vi "Spawn.vi"(6 "Start Direction":T1=enum."E", 8 "error in (no error)":errorcluster, 10 "Directive":T2, 11 "Mother in":refnum<class "Formics.lvclass">) -> (0 "error out":errorcluster, 2 "Replicated Class":refnum<class "Formics.lvclass">, 3 "Mother out":refnum<class "Formics.lvclass">)   [LabVIEW 2015, in "Formics.lvclass"]
uses:
  Formics.lvclass
  Formic Types.ctl
  Type Defs/Direction Enum.ctl
  Current Directive.ctl
  Formics.lvclass/Formics.ctl
  Coward Options.ctl
  Type Defs/SB Type Defs.lvlib
panel:
  in  "Spawn Direction":T1=enum."E"
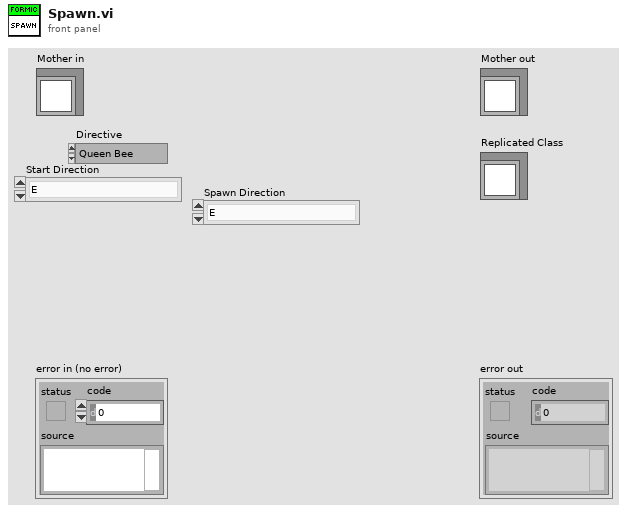
[diagram p1: front panel]
types:
  T1 = typedef "SB Type Defs.lvlib/Direction Enum.ctl" = enum16{"NW", "N", "NE", "E", "SE", "S", "SW", "W"}
  T2 = typedef "Formics.lvclass/Formic Types.ctl" = enum16{"Queen Bee", "Protector Bee", "Daughter Bee", "Worker Bee", "Coward"}
  T3 = typedef "Formics.lvclass/Current Directive.ctl" = enum16{"Queen", "Daughter", "Coward", "Migrate", "Line Up", "Protector", "Scout"}
  T4 = typedef "Formics.lvclass/Coward Options.ctl" = enum16{"Go", "Attack behind and continue", "Attack behind and recheck", "Move Back", "Check if still there"}
  T5 = typedef "Formics.lvclass/SquareStatus DVR.ctl" = refnum<data-value>
  T6 = typedef "Formics.lvclass/Kamikaze DVR.ctl" = refnum<data-value>
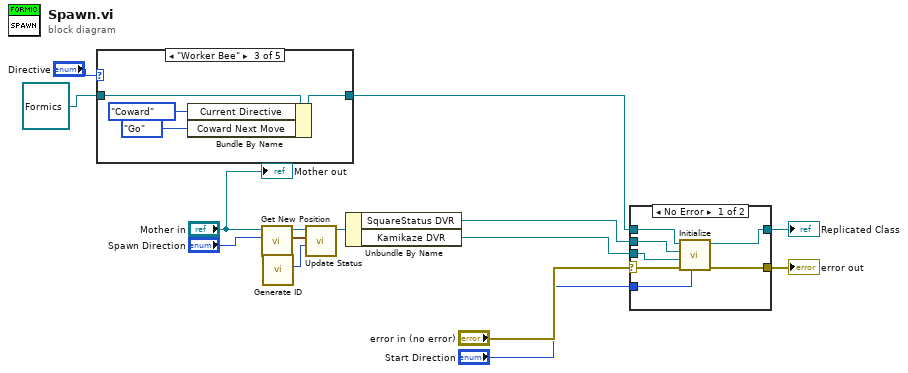
[diagram p0: block diagram]
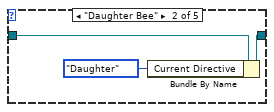
[diagram p3: hidden frame]
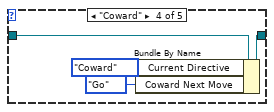
[diagram p4: hidden frame]
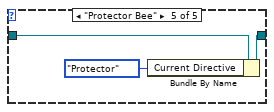
[diagram p5: hidden frame]
diagram:
  n1 = case shown="\"Worker Bee\"" "Directive" {
    tunnel: [w16 w19 w22 w27 w30] -> w12
    tunnel: refnum<class "Formics.lvclass"> refnum ("Formics.lvclass") -> [w16 w18 w23 w25 w28]
    frame "Queen Bee", Default {
    }
    frame "Daughter Bee" {
      n2 = Bundle By Name(cluster=w18, "Current Directive"=Current_Directive."Daughter") -> (w19:refnum<class "Formics.lvclass">)
    }
    frame "Worker Bee" {
      n3 = Bundle By Name(cluster=w23, "Current Directive"=Current_Directive."Coward", "Coward Next Move"=Coward_Options."Go" ("Next Move")) -> (w22:refnum<class "Formics.lvclass">)
    }
    frame "Coward" {
      n4 = Bundle By Name(cluster=w25, "Current Directive"=Current_Directive."Coward", "Coward Next Move"=Coward_Options."Go" ("Next Move")) -> (w27:refnum<class "Formics.lvclass">)
    }
    frame "Protector Bee" {
      n5 = Bundle By Name(cluster=w28, "Current Directive"=Current_Directive."Protector") -> (w30:refnum<class "Formics.lvclass">)
    }
  }
  n6 = call "Get New Position.vi"("Direction"="Spawn Direction", "Formics in"="Mother in") -> ("MyPosition"=w4:cluster{"X":i32, "Y":i32}, "Formics out"=w2:refnum<class "Formics.lvclass">)  [unwired: 8 in]
  n7 = call "Generate ID.vi"() -> ("Unique ID"=w7:i32)  [unwired: 11 in]
  n8 = call "Update Status.vi"("ID"=w7, "MyPosition"=w4, "Mother in"=w2) -> ("Mother out"=w6:refnum<class "Formics.lvclass">)  [unwired: 8 in]
  n9 = Unbundle By Name(w6) -> ("SquareStatus DVR"=w8:T5, "Kamikaze DVR"=w10:T6)
  n10 = case shown="No Error" "error in (no error)" {
    selector: "error in (no error)" -> [w37 w39]
    tunnel: [w36 w39] -> w14
    tunnel: [w34 w38] -> w11
    tunnel: w12 -> [w35 w38]
    tunnel: w8 -> [w33 _]
    tunnel: w10 -> [w32 _]
    tunnel: "Start Direction" -> [w31 _]
    frame No Error {
      n11 = call-dynamic "Initialize.vi"("Start Direction"=w31, "error in (no error)"=w37, "Kamikaze DVR"=w32, "SquareStatus DVR"=w33, "Mother in"=w35) -> ("error out"=w36:errorcluster, "Mother out"=w34:refnum<class "Formics.lvclass">)  [unwired: 5 in]
    }
    frame Error {
    }
  }
  "error out" <- w14
  "Replicated Class" <- w11
  "Mother out" <- "Mother in"
